vi "Send New Parameter.vi"(8 "error in (no error)":errorcluster, 10 "New parameter":variant, 11 "controller in":refnum<class "Generic Plugin.lvclass">) -> (0 "error out":errorcluster, 3 "controller out":refnum<class "Generic Plugin.lvclass">)   [LabVIEW 2020, in "RxnRover.lvlib" / "Generic Plugin.lvclass"]
doc: "Sends the new set of parameters to the associated plugin."
uses:
  Generic Plugin.lvclass
  Generic Plugin.lvclass/Generic Plugin.ctl
  <userlib>/RxnRover/DynamicReentrant/Dynamic Reentrant.lvlib
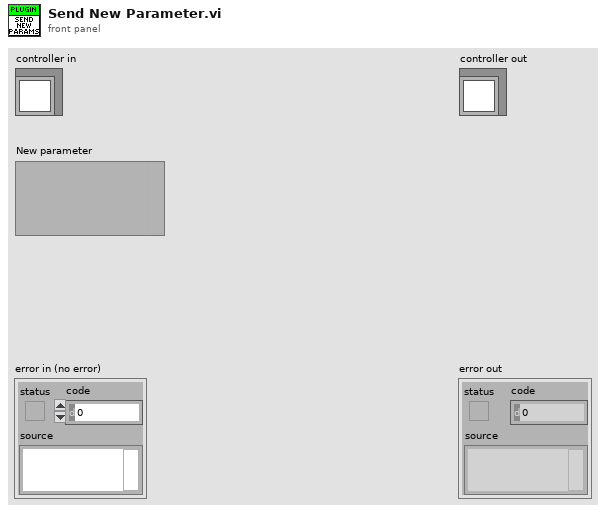
[diagram p1: front panel]
types:
  T1 = typedef "Dynamic Reentrant.lvlib/Message.ctl" = cluster{"Source":string, "Destination":string, "Time Stamp":timestamp, "Command":string, "Data":variant}
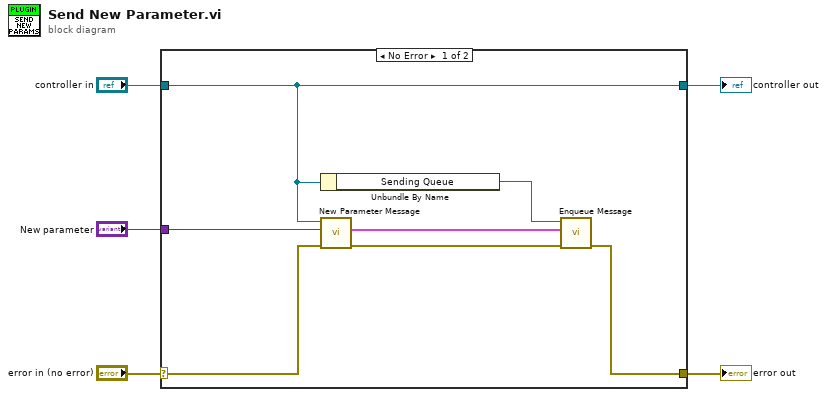
[diagram p0: block diagram]
diagram:
  n1 = case shown="No Error" "error in (no error)" {
    selector: "error in (no error)" -> [w8 w14]
    tunnel: [w6 w14] -> w4
    tunnel: [w11 w13] -> w2
    tunnel: "controller in" -> [w11 w13]
    tunnel: "New parameter" -> [w7 _]
    frame No Error {
      n2 = Unbundle By Name(w11) -> ("Sending Queue"=w12:refnum<queue>)
      n3 = call-dynamic "New Parameter Message.vi"("error in (no error)"=w8, "New parameter"=w7, "Generic Controller in"=w11) -> ("error out"=w9:errorcluster, "New Parameter Message"=w10:T1)  [unwired: 6 in, 1 out]
      n4 = call <userlib>:"Enqueue Message.vi"("error in (no error)"=w9, "Message"=w10, "Listening Queue"=w12) -> ("error out"=w6:errorcluster)  [unwired: 7 in, 1 out]
    }
    frame Error {
    }
  }
  "error out" <- w4
  "controller out" <- w2
